vi "AuMT8852B EDR CW Measurement Configuration.vi"(5 "Settings":T2={"Modulation Scheme (PI4)"=enum."PI4", "Frequency (2402)"=2402.0, "Frequency units (MHz)"=enum."MHz", "Gate width (1 ms)"=1.0} {"Gate width (1 ms)" format="%.2f"}, 7 "Set/Get (Set)":enum16{"Set", "Get"}(ring), 8 "error in (no error)":errorcluster, 11 "VISA session":refnum<visa-resource-name>) -> (0 "error out":errorcluster, 2 "error code":i32, 3 "VISA session out":refnum<visa-resource-name>, 4 "Settings out":T1={"Modulation Scheme"=enum."PI4", "Frequency"=2441.0, "Frequency units"=enum."MHz", "Gate width"=1.0} {"Gate width" format="%.2f"})   [LabVIEW 2017]
doc: "Anritsu MT8852B Bluetooth Tester\n\nPlaces the instrument into EDR CW measurement mode and sets the modulation scheme, the frequency channel and the gate width for power and DEVM measurements.\n\nINPUTS\nSet/Get - whether the configuration is being sent to or retrieved from the instrument.\n(Settings)\nModulation Scheme - the EDR modulation scheme used in the test.\nFrequency units - whether frequency will be read/written as a channel or as a frequency in MHz. \nFrequency - frequency at which the ECW measurement will be made.\nGate width - measurement period (0.1 to 3.0) in ms.\n\nOUTPUTS\n(Settings out)\nModulation Scheme - the current EDR modulation scheme used in the test.\nFrequency units out - whether frequency is returned as a channel or as a frequency in MHz.\nFrequency out - current ECW measurement frequency.\nGate width - current CW measurement period in ms."
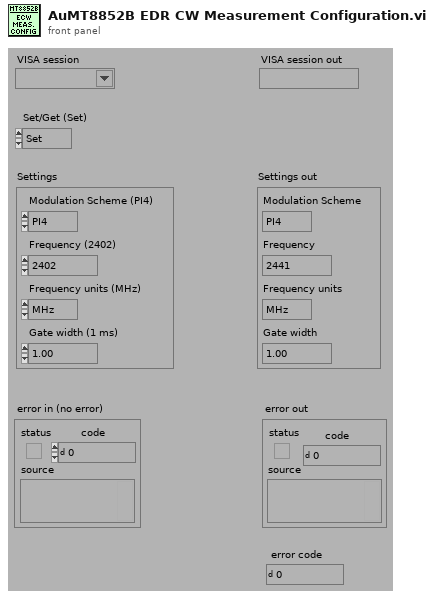
[diagram p1: front panel]
types:
  T1 = cluster{"Modulation Scheme":enum16{"PI4", "8DPSK"}, "Frequency":dbl, "Frequency units":enum16{"Channel", "MHz"}, "Gate width":dbl}
  T2 = cluster{"Modulation Scheme (PI4)":enum16{"PI4", "8DPSK"}, "Frequency (2402)":dbl, "Frequency units (MHz)":enum16{"Channel", "MHz"}, "Gate width (1 ms)":dbl}
  T3 = enum16{"Simulate", "Range check", "Cache", "Query instrument status"}
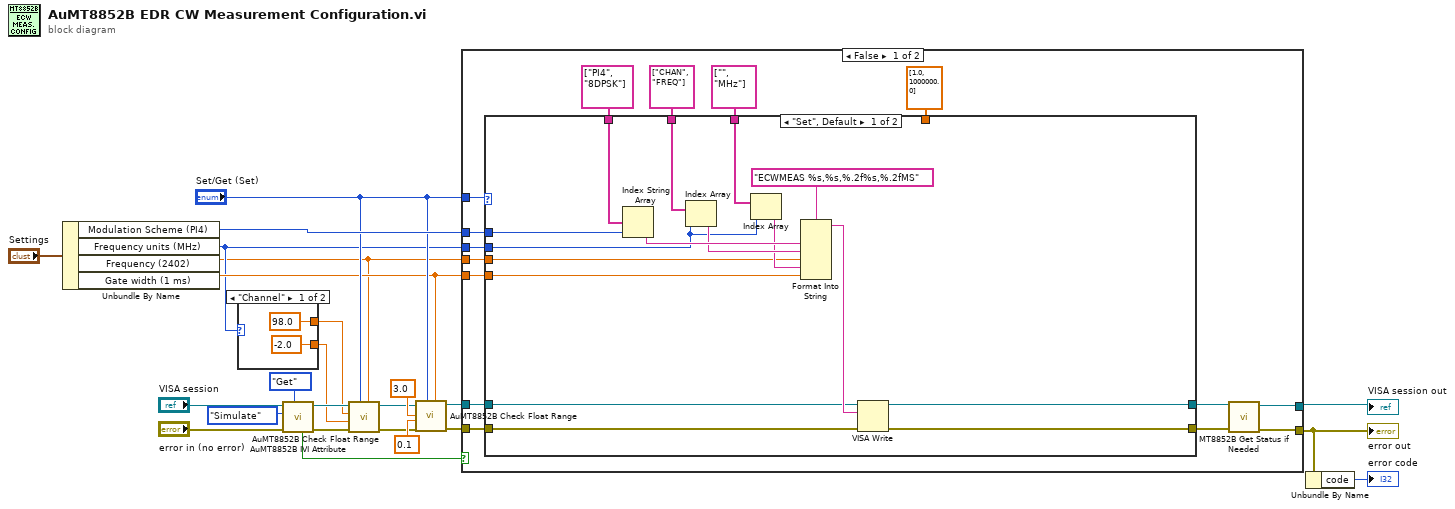
[diagram p0: block diagram]
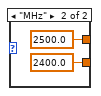
[diagram p2: hidden frame]
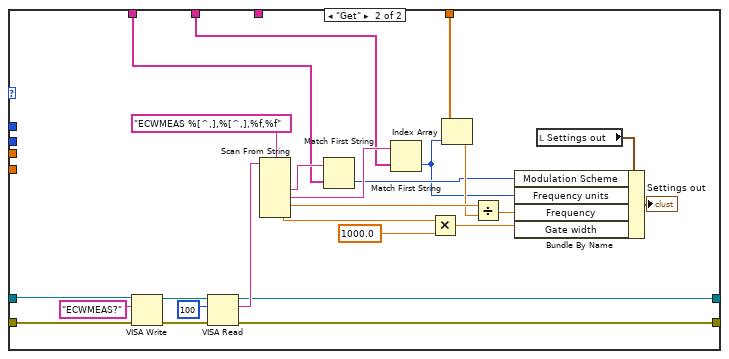
[diagram p3: hidden frame]
diagram:
  n1 = Unbundle By Name("Settings") -> ("Modulation Scheme (PI4)"=w11:enum16{"PI4", "8DPSK"}, "Frequency units (MHz)"=w2:enum16{"Channel", "MHz"}, "Frequency (2402)"=w1:dbl, "Gate width (1 ms)"=w5:dbl)
  n2 = case shown="\"Channel\"" w2 {
    tunnel: [98.0 ("Upper limit (1)") 2500.0 ("Upper limit (1)")] -> w4
    tunnel: [-2.0 ("Lower limit (-1)") 2400.0 ("Lower limit (-1)")] -> w3
    frame "Channel" {
    }
    frame "MHz" {
    }
  }
  n3 = call <instrlib>:"AuMT8852B IVI Attribute.vi"("Set/Get (Set)"=enum16{"Set", "Get"}."Get", "error in (no error)"="error in (no error)", "Flag (Simulate)"=T3."Simulate", "VISA session"="VISA session") -> ("error out"=w20:errorcluster, "VISA session out"=w19:refnum<visa-resource-name>, "Value out"=w14:bool)  [unwired: 5 in]
  n4 = call <instrlib>:"AuMT8852B Check Float Range.vi"("Value (0)"=w1, "Set/Get (Set)"="Set/Get (Set)", "error in (no error)"=w20, "Lower limit (-1)"=w3, "Upper limit (1)"=w4, "VISA session"=w19) -> ("error out"=w15:errorcluster, "VISA session out"=w16:refnum<visa-resource-name>)  [unwired: 4 in]
  n5 = call <instrlib>:"AuMT8852B Check Float Range.vi"("Value (0)"=w5, "Set/Get (Set)"="Set/Get (Set)", "error in (no error)"=w15, "Lower limit (-1)"=0.1, "Upper limit (1)"=3.0, "VISA session"=w16) -> ("error out"=w13:errorcluster, "VISA session out"=w12:refnum<visa-resource-name>)  [unwired: 4 in]
  n6 = case shown="False" w14 {
    tunnel: [w29 w86] -> w7
    tunnel: [w30 w85] -> w8
    tunnel: w13 -> [w38 w85]
    tunnel: w12 -> [w37 w86]
    tunnel: w1 -> [w36 _]
    tunnel: "Set/Get (Set)" -> [w35 _]
    tunnel: w11 -> [w34 _]
    tunnel: w2 -> [w33 _]
    tunnel: w5 -> [w32 _]
    frame False {
      n7 = case shown="\"Set\", Default" w35 {
        tunnel: [w59 w78] -> w39
        tunnel: [w58 w77] -> w40
        tunnel: string[] ["PI4", "8DPSK"] -> [w50 w67]
        tunnel: string[] ["CHAN", "FREQ"] ("Array Constant") -> [w52 w66]
        tunnel: string[] ["", "MHz"] ("Array Constant") -> [w53 _]
        tunnel: dbl[] [1.0, 1000000.0] ("Array Constant") -> [_ w76]
        tunnel: w38 -> [w55 w75]
        tunnel: w37 -> [w54 w74]
        tunnel: w36 -> [w46 _]
        tunnel: w34 -> [w44 _]
        tunnel: w33 -> [w45 _]
        tunnel: w32 -> [w47 _]
        frame "Set", Default {
          n8 = Index String Array(1:w44, 2:w50) -> (0:w51:string)  [unwired: 1 in]
          n9 = Index Array(array=w52, index=w45) -> (element=w49:string)
          n10 = Index Array(array=w53, index=w45) -> (element=w48:string)
          n11 = Format Into String(format string="ECWMEAS %s,%s,%.2f%s,%.2fMS" ("Format String"), w51, w49, w46, w48, w47) -> (resulting string=w56:string)  [unwired: 2 in, 1 out]
          n12 = VISA Write(VISA resource name=w54, write buffer=w56, error in (no error)=w55) -> (VISA resource name out=w59:refnum<visa-resource-name>, error out=w58:errorcluster)  [unwired: 1 out]
        }
        frame "Get" {
          n13 = VISA Write(VISA resource name=w74, write buffer="ECWMEAS?" ("write buffer (\"\")"), error in (no error)=w75) -> (VISA resource name out=w81:refnum<visa-resource-name>, error out=w82:errorcluster)  [unwired: 1 out]
          n14 = VISA Read(VISA resource name=w81, byte count=u32 100 ("byte count (0)"), error in (no error)=w82) -> (VISA resource name out=w78:refnum<visa-resource-name>, read buffer=w79:string, error out=w77:errorcluster)  [unwired: 1 out]
          n15 = Scan From String(format string="ECWMEAS %[^,],%[^,],%f,%f" ("Format String"), input string=w79) -> (output 1=w69:string, output 2=w68:string, output 3=w71:dbl, output 4=w73:dbl)  [unwired: 6 in, 3 out]
          n16 = Match First String(2:w67, 3:w69) -> (0:w63:i32)  [unwired: 1 out]
          n17 = Match First String(2:w66, 3:w68) -> (0:w60:i32)  [unwired: 1 out]
          n18 = Multiply(x=w73, y=1000.0) -> (x*y=w65:dbl)
          n19 = Index Array(array=w76, index=w60) -> (element=w70:dbl)
          n20 = Divide(x=w71, y=w70) -> (x/y=w64:dbl)
          n21 = local read "Settings out"() -> (w61:T1)
          n22 = Bundle By Name(cluster=w61, "Modulation Scheme"=w63, "Frequency units"=w60, "Frequency"=w64, "Gate width"=w65) -> (→"Settings out":T1)
        }
      }
      n23 = call <instrlib>:"MT8852B Get Status if Needed.vi"("error in (no error)"=w40, "VISA session"=w39) -> ("error out"=w30:errorcluster, "VISA session out"=w29:refnum<visa-resource-name>)  [unwired: 8 in]
    }
    frame True {
    }
  }
  "error out" <- w8
  "VISA session out" <- w7
  n24 = Unbundle By Name(w8) -> ("code"=→"error code":i32)
